vi "Polarímetro.vi"() -> ()   [LabVIEW 2024]
uses:
  <instrlib>/Arduino UNO/Arduino UNO.lvlib
panel:
  out "Loop":i32
  out "XY Graph":cluster{"Y":dbl[], "Y":dbl[]}[](graph)
  in  "VISA resource name":refnum<visa-resource-name>
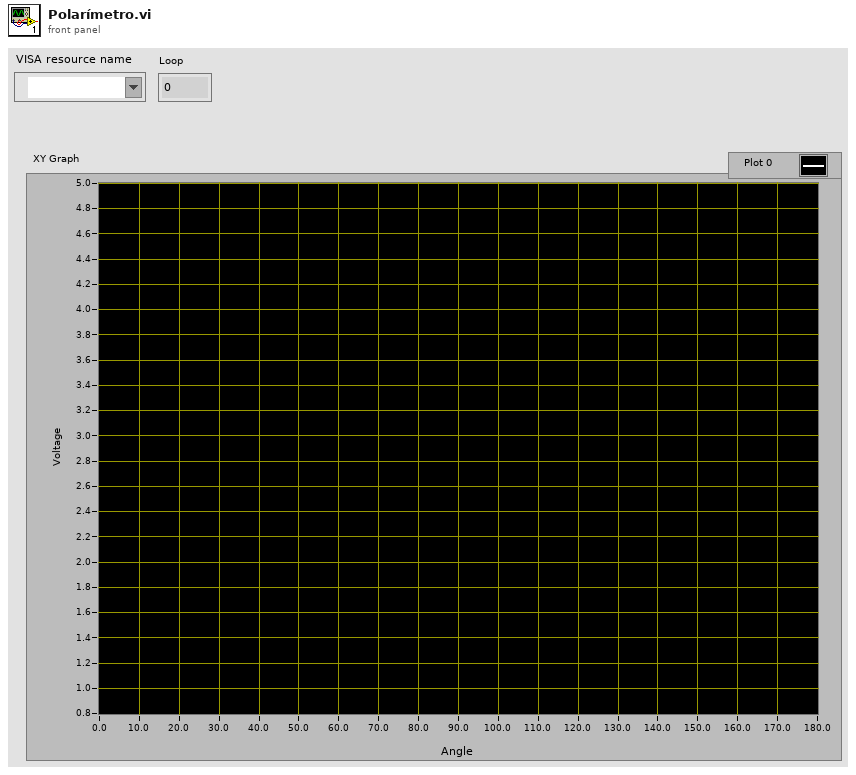
[diagram p1: front panel]
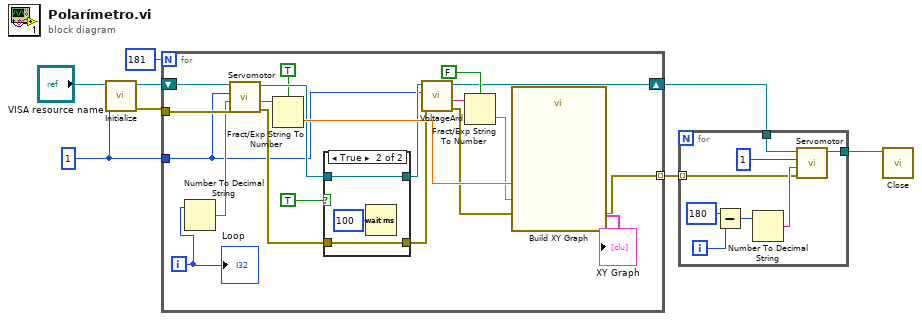
[diagram p0: block diagram]
diagram:
  w7 = u8 1 ("Address")
  n1 = call <instrlib>:"Initialize.vi"("Address"=w7, "VISA resource name"="VISA resource name") -> ("error IO"=w6:errorcluster, "VISA resource name out"=w5:refnum<visa-resource-name>)  [unwired: 7 in, 1 out]
  n2 = for {
    N: 181 -> [_]
    tunnel: w7 -> [w10]
    tunnel: w6 -> [w27]
    shift-right: [w13] -> w3
    shift-left: w5 -> [w26]
    tunnel: [w12] -> w1 mode=indexing
    i -> [w22]
    n3 = Number To Decimal String(number=w22) -> (decimal integer string=w23:string)  [unwired: 1 in]
    n4 = call <instrlib>:"Servomotor.vi"("error in (no error)"=w27, "Data"=w23, "Address"=w10, "VISA resource name"=w26) -> ("error IO"=w17:errorcluster, "Angle"=w24:string, "VISA resource name out"=w18:refnum<visa-resource-name>)  [unwired: 5 in]
    n5 = Fract/Exp String To Number(use system decimal point (T)=TRUE, string=w24) -> (number=w21:dbl)  [unwired: 2 in, 1 out]
    n6 = case shown="True" TRUE {
      tunnel: [w29 w32] -> w14
      tunnel: w18 -> [w29 w32]
      tunnel: [w28 w30] -> w11
      tunnel: w17 -> [w28 w30]
      frame False {
      }
      frame True {
        n7 = Wait (ms)(milliseconds to wait=u32 100) -> ()  [unwired: 1 out]
      }
    }
    n8 = call <instrlib>:"VoltageArd.vi"("error in (no error)"=w11, "Address"=w10, "VISA resource name"=w14) -> ("error IO"=w12:errorcluster, "Voltage"=w9:string, "VISA resource name out"=w13:refnum<visa-resource-name>)  [unwired: 6 in]
    n9 = Fract/Exp String To Number(use system decimal point (T)=FALSE, string=w9) -> (number=w20:dbl)  [unwired: 2 in, 1 out]
    n10 = call "Build XY Graph"("Y Input"=w20, "X Input"=w21) -> ("XY Graph"=→"XY Graph":cluster{"X":dbl[], "Y":dbl[]}[])  [unwired: 8 in, 1 out]
    "Loop" <- w22
  }
  n11 = for {
    tunnel: w3 -> [w35]
    tunnel: [w34] -> w2
    tunnel: w1 -> [w33] mode=indexing
    i -> [w40]
    n12 = Subtract(x=180, y=w40) -> (x-y=w38:i32)
    n13 = Number To Decimal String(number=w38) -> (decimal integer string=w37:string)  [unwired: 1 in]
    n14 = call <instrlib>:"Servomotor.vi"("error in (no error)"=w33, "Data"=w37, "Address"=u8 1, "VISA resource name"=w35) -> ("VISA resource name out"=w34:refnum<visa-resource-name>)  [unwired: 5 in, 2 out]
  }
  n15 = call <instrlib>:"Close.vi"("VISA resource name"=w2) -> ()  [unwired: 10 in, 1 out]
